vi "Introspection Core.vi"(8 "error in (no error)":errorcluster, 11 "BNT_DAQmx-MCSV in":refnum<class "BNT_DAQmx-MCSV.lvclass">) -> (0 "error out":errorcluster, 1 "CSPPMessages":refnum<class "Message.lvclass">[](array[class]), 2 "Class History":string[](array[string]), 3 "BNT_DAQmx-MCSV out":refnum<class "BNT_DAQmx-MCSV.lvclass">)   [LabVIEW 2020, in "BNT_DAQmx.lvlib" / "BNT_DAQmx-MCSV.lvclass"]
doc: "This vi delivers a list with all messages this actor reacts to. \n\nNote that all inherited classes have to overwrite it."
uses:
  BNT_DAQmx-MCSV.lvclass
  <vilib>/ActorFramework/Message/Message.lvclass
  BNT_DAQmx-MCSV Messages/Readout Msg/Readout Msg.lvclass
  C:/Program Files (x86)/National Instruments/LabVIEW 2020/vi.lib/ActorFramework/Message/Message.lvclass
  BNT_DAQmx-MCSV Messages/Set Output Lines Msg/Set Output Lines Msg.lvclass
  BNT_DAQmx-MCSV Messages/Set Output Line Msg/Set Output Line Msg.lvclass
  BNT_DAQmx-MCSV Messages/Set Output Value Msg/Set Output Value Msg.lvclass
  BNT_DAQmx-MCSV Messages/Set Output Values Msg/Set Output Values Msg.lvclass
  CSPP_Core/Actors/CSPP_DeviceActor/CSPP_DeviceActor.lvclass
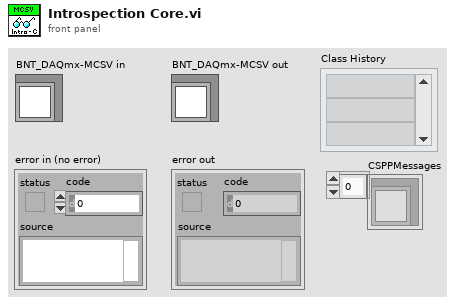
[diagram p1: front panel]
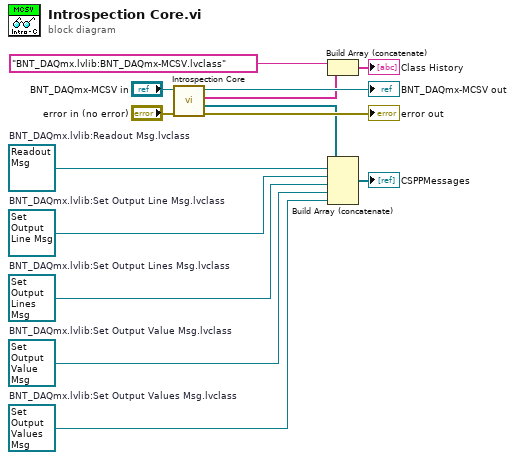
[diagram p0: block diagram]
diagram:
  w5 = refnum<class "Set Output Values Msg.lvclass"> refnum  # BNT_DAQmx.lvlib:Set Output Values Msg.lvclass
  w6 = refnum<class "Set Output Value Msg.lvclass"> refnum  # BNT_DAQmx.lvlib:Set Output Value Msg.lvclass
  w7 = refnum<class "Set Output Line Msg.lvclass"> refnum  # BNT_DAQmx.lvlib:Set Output Line Msg.lvclass
  w8 = refnum<class "Set Output Lines Msg.lvclass"> refnum  # BNT_DAQmx.lvlib:Set Output Lines Msg.lvclass
  w9 = refnum<class "Readout Msg.lvclass"> refnum  # BNT_DAQmx.lvlib:Readout Msg.lvclass
  n1 = call-parent "Introspection Core.vi"("Error In"="error in (no error)", "CSPP_DeviceActor in"="BNT_DAQmx-MCSV in") -> ("Error Out"=→"error out":errorcluster, "CSPP_Messages"=w4:refnum<class "Message.lvclass">[], "Class History"=w2:string[], "CSPP_DeviceActor out"=→"BNT_DAQmx-MCSV out":refnum<class "BNT_DAQmx-MCSV.lvclass">)  [unwired: 6 in]
  n2 = Build Array (concatenate)("BNT_DAQmx.lvlib:BNT_DAQmx-MCSV.lvclass", w2) -> (→"Class History":string[])
  n3 = Build Array (concatenate)(w4, w9, w7, w8, w6, w5) -> (→"CSPPMessages":refnum<class "Message.lvclass">[])
